vi "IntakeNetwork_ReadSlow.vi"(8 "error in (no error)":errorcluster) -> (0 "error out":errorcluster)   [LabVIEW 2023]
uses:
  <vilib>/Rock Robotics/Network Tables/NT Get Topic.vi
  <vilib>/Rock Robotics/Network Tables/NT Get PublishHandle.vi
  <vilib>/Rock Robotics/Network Tables/NT_LL_Write Boolean.vi
  <vilib>/Rock Robotics/Network Tables/NT Check Errors.vi
  <vilib>/Rock Robotics/Network Tables/NT Read Number.vi
  <vilib>/Rock Robotics/Network Tables/NT_LL_Write Number.vi
  IntakeGlobal.vi
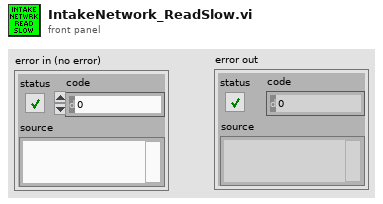
[diagram p1: front panel]
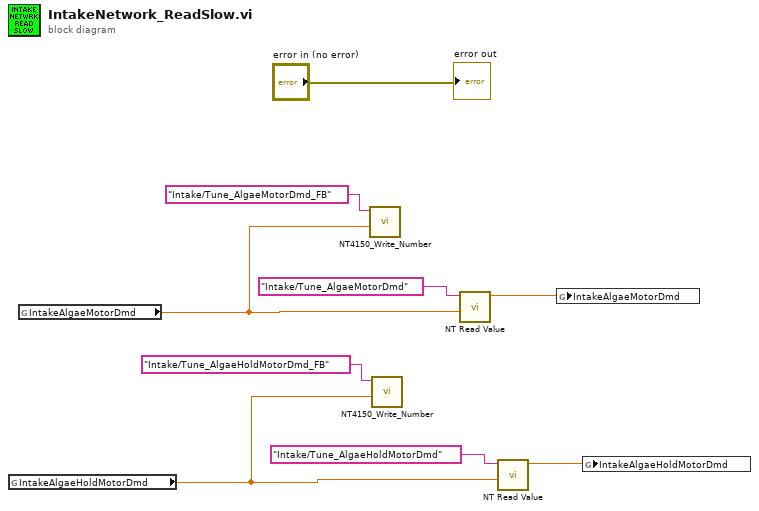
[diagram p0: block diagram]
diagram:
  n1 = global read "IntakeGlobal.vi" "IntakeAlgaeHoldMotorDmd"() -> (w1:dbl)
  n2 = global read "IntakeGlobal.vi" "IntakeAlgaeMotorDmd"() -> (w5:dbl)
  n3 = call "NT4150_Write_Number.vi"("value"=w5, "name"="Intake/Tune_AlgaeMotorDmd_FB") -> ()  [unwired: 9 in, 1 out]
  n4 = call "NT4150_Write_Number.vi"("value"=w1, "name"="Intake/Tune_AlgaeHoldMotorDmd_FB") -> ()  [unwired: 9 in, 1 out]
  n5 = call-poly <vilib>:"NT Read Value.vi"("default value"=w5, "name"="Intake/Tune_AlgaeMotorDmd") -> ("value"=w6:dbl)  [unwired: 7 in, 2 out]
  n6 = call-poly <vilib>:"NT Read Value.vi"("default value"=w1, "name"="Intake/Tune_AlgaeHoldMotorDmd") -> ("value"=w2:dbl)  [unwired: 7 in, 2 out]
  n7 = global write "IntakeGlobal.vi" "IntakeAlgaeMotorDmd"(w6) -> ()
  n8 = global write "IntakeGlobal.vi" "IntakeAlgaeHoldMotorDmd"(w2) -> ()
  "error out" <- "error in (no error)"
